vi "Read status.vi"(8 "error in (no error)":errorcluster, 11 "_ISerializable in":refnum<class "_ISerializable.lvclass">) -> (0 "error out":errorcluster, 2 "status":u8, 3 "_ISerializable out":refnum<class "_ISerializable.lvclass">)   [LabVIEW 2018, in "_ISerializable.lvclass"]
uses:
  _ISerializable.lvclass
  _ISerializable.lvclass/_ISerializable.ctl
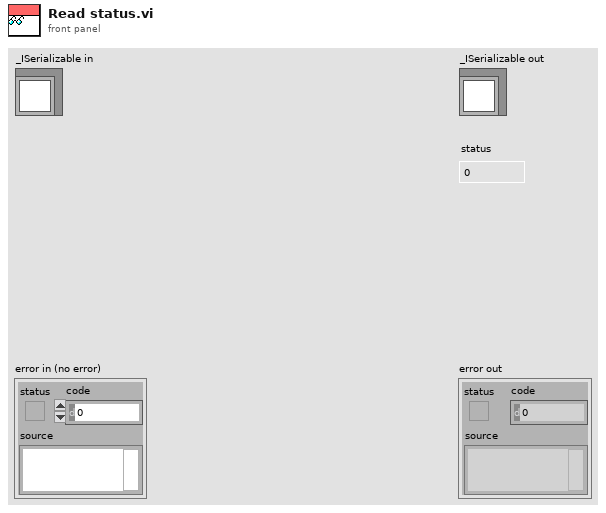
[diagram p1: front panel]
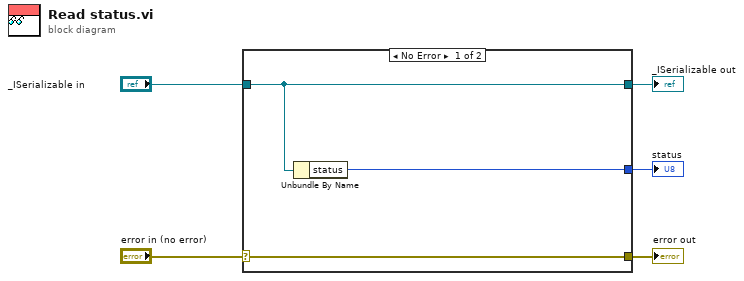
[diagram p0: block diagram]
diagram:
  n1 = case shown="No Error" "error in (no error)" {
    selector: "error in (no error)" -> [w8 w9]
    tunnel: [w8 w9] -> w4
    tunnel: [w7 w10] -> w2
    tunnel: "_ISerializable in" -> [w7 w10]
    tunnel: [w6 _] -> w1
    frame No Error {
      n2 = Unbundle By Name(w7) -> ("status"=w6:u8)
    }
    frame Error {
    }
  }
  "error out" <- w4
  "_ISerializable out" <- w2
  "status" <- w1
